vi "Calculate Recovery Time.vi"(8 "Error In":errorcluster, 11 "110-130 Array":dbl[][](array[numeric])) -> (0 "Error Out":errorcluster, 2 "No Data Found Between 110-130":bool, 3 "HP Recovery Time":dbl format="%#.4g")   [LabVIEW 2019]
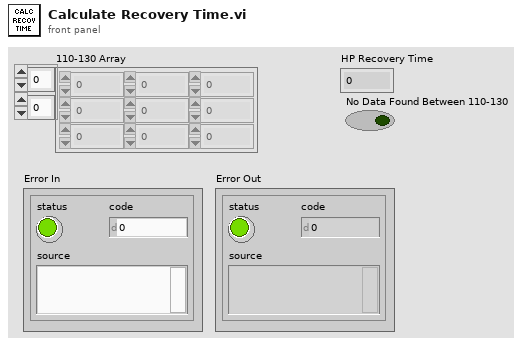
[diagram p1: front panel]
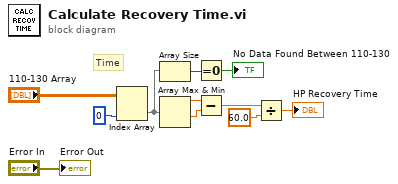
[diagram p0: block diagram]
diagram:
  # "Time"
  n1 = Index Array(array="110-130 Array", index (col)=0 ("disabled index (col)")) -> (element=w8:dbl[])  [unwired: 1 in]
  n2 = Array Size(array=w8) -> (size(s)=w9:i32)
  n3 = Array Max & Min(array=w8) -> (max value=w3:dbl, min value=w4:dbl)  [unwired: 2 out]
  n4 = Equal To 0?(x=w9) -> (x = 0?=→"No Data Found Between 110-130":bool)
  n5 = Subtract(x=w3, y=w4) -> (x-y=w5:dbl)
  n6 = Divide(x=w5, y=60.0) -> (x/y=→"HP Recovery Time":dbl)
  "Error Out" <- "Error In"
